vi "Build Driver Settings Mappings.vi"(8 "error in (no error)":errorcluster, 11 "SDS1104X-E in":refnum<class "SDS1104X-E.lvclass">) -> (0 "error out":errorcluster, 2 "Array":T1[](array[typedef]), 3 "SDS1104X-E out":refnum<class "SDS1104X-E.lvclass">)   [LabVIEW 2023, in "HAF.lvlib" / "SDS1104X-E.lvclass"]
doc: "The SDS1104X-E has no Driver Settings so build an empty array."
uses:
  SDS1104X-E.lvclass
  SDS1104X-E.lvclass/SDS1104X-E.ctl
  Setting Map Structure.ctl
  HAF.lvlib
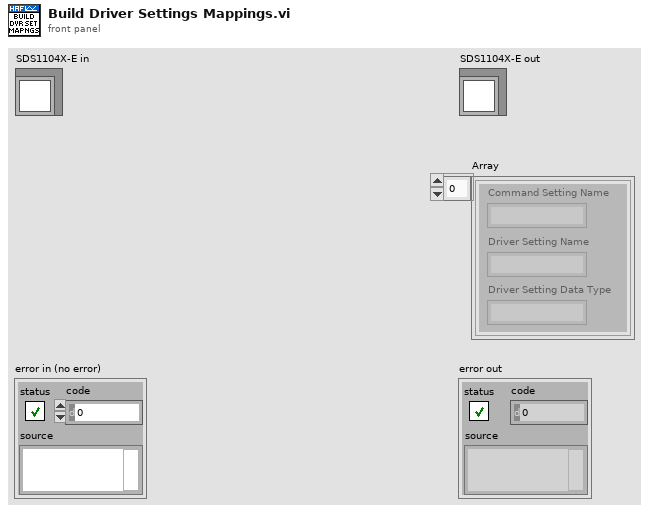
[diagram p1: front panel]
types:
  T1 = typedef "HAF.lvlib/Setting Map Structure.ctl" = cluster{"Command Setting Name":string, "Driver Setting Name":string, "Driver Setting Data Type":string}
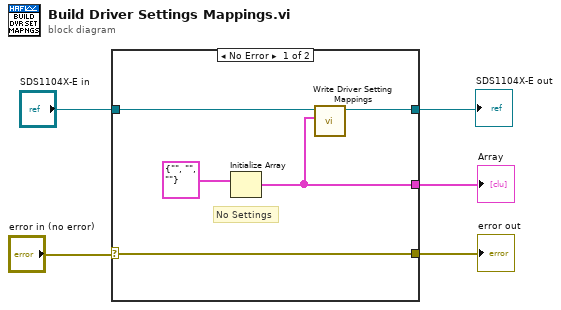
[diagram p0: block diagram]
diagram:
  n1 = case shown="No Error" "error in (no error)" {
    selector: "error in (no error)" -> [w6 w11]
    tunnel: [w8 _] -> w2
    tunnel: "SDS1104X-E in" -> [w9 w12]
    tunnel: [w7 w12] -> w3
    tunnel: [w6 w11] -> w1
    frame No Error {
      # "No Settings"
      n2 = Initialize Array(T1 {"Command Setting Name"="", "Driver Setting Name"="", "Driver Setting Data Type"=""} ("Mapping")) -> (w8:T1[])  [unwired: 1 in]
      n3 = call-dynamic "Write Driver Setting Mappings.vi"("Driver Setting Mappings"=w8, "Driver in"=w9) -> ("Driver out"=w7:refnum<class "SDS1104X-E.lvclass">)  [unwired: 8 in, 1 out]
    }
    frame Error {
    }
  }
  "error out" <- w1
  "SDS1104X-E out" <- w3
  "Array" <- w2
